vi "ExamplePluginOOBService ExportPath.vi"(6 "contextId":T1, 8 "error in":errorcluster, 9 "timeout (ms)":i32=-1, 10 "Request Data":T3, 11 "gRPC ID":T1) -> (0 "error out":errorcluster, 2 "Response Data":T2, 3 "gRPC ID out":T1)   [LabVIEW 2025, in "Automotive-Vision-OOBService_client.lvlib"]
uses:
  Automotive-Vision-OOBService_client.lvlib
  <vilib>/gRPC/LabVIEW gRPC Library/Shared/grpcId.ctl
  RPC Messages/hwval_ExportRequest.ctl
  RPC Messages/hwval_StatusResponse.ctl
  RPC Messages/hwval_StatusResponse_Flat.ctl
  14035477-4c25-4107-8ed5-d0c4ef420ce5.vi
  <vilib>/gRPC/LabVIEW gRPC Library/Shared/TranslateGrpcError.vi
  <vilib>/gRPC/LabVIEW gRPC Library/Shared/Wait On Occurrence.vi
  <vilib>/gRPC/LabVIEW gRPC Library/Shared/Is Feature Enabled.vi
  <vilib>/gRPC/LabVIEW gRPC Library/Server API/Server/Get Server DLL Path.vi
  <vilib>/Utility/error.llb/Error Cluster From Error Code.vi
  <vilib>/gRPC/LabVIEW gRPC Library/grpc-lvsupport-release.lvlib
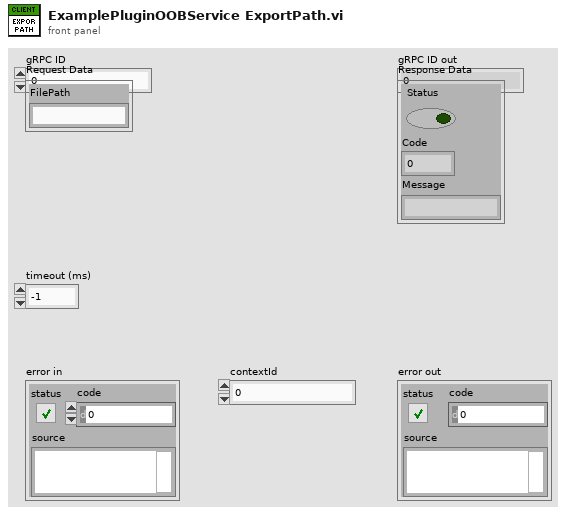
[diagram p1: front panel]
types:
  T1 = typedef "grpc-lvsupport-release.lvlib/grpcId.ctl" = u64
  T2 = typedef "Automotive-Vision-OOBService_client.lvlib/hwval_StatusResponse.ctl" = cluster{"Status":bool, "Code":i32, "Message":string}
  T3 = typedef "Automotive-Vision-OOBService_client.lvlib/hwval_ExportRequest.ctl" = cluster{"FilePath":string}
  T4 = typedef "Automotive-Vision-OOBService_client.lvlib/hwval_StatusResponse_Flat.ctl" = cluster{"Status":bool, "Code":i32, "Message":string}
  T5 = typedef "Automotive-Vision-OOBService_client.lvlib/hwval_ExportRequest_Flat.ctl" = cluster{"FilePath":string}
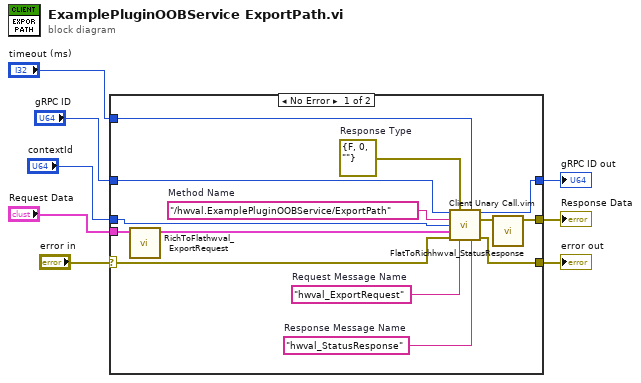
[diagram p0: block diagram]
diagram:
  n1 = case shown="No Error" "error in" {
    selector: "error in" -> [w18 w23]
    tunnel: [w17 w23] -> w7
    tunnel: "gRPC ID" -> [w16 w24]
    tunnel: [w15 w24] -> w5
    tunnel: "Request Data" -> [w12 _]
    tunnel: [w9 _] -> w3
    tunnel: "timeout (ms)" -> [w14 _]
    tunnel: "contextId" -> [w13 _]
    frame No Error {
      w19 = "hwval_StatusResponse"  # Response Message Name
      w20 = "hwval_ExportRequest"  # Request Message Name
      w21 = T4 {"Status"=FALSE, "Code"=0, "Message"=""}  # Response Type
      w22 = "/hwval.ExamplePluginOOBService/ExportPath"  # Method Name
      n2 = call "RichToFlathwval_ExportRequest.vi"("InputCluster"=w12) -> ("OutputCluster"=w11:T5)  [unwired: 10 in]
      n3 = call "Client Unary Call.vim"("ClientID in"=w16, "Response Type"=w21, "timeout (ms)"=w14, "Method Name"=w22, "contextId"=w13, "Request Data"=w11, "error in"=w18, "Request Message Name"=w20, "Response Message Name"=w19) -> ("ClientID out"=w15:u64, "Response Data"=w10:T4, "error out"=w17:errorcluster)  [unwired: 4 in]
      n4 = call "FlatToRichhwval_StatusResponse.vi"("InputCluster"=w10) -> ("OutputCluster"=w9:T2)  [unwired: 10 in]
    }
    frame Error {
    }
  }
  "error out" <- w7
  "gRPC ID out" <- w5
  "Response Data" <- w3
